vi "main.vi"() -> ()   [LabVIEW 2024]
uses:
  main_state.ctl
  server_state.ctl
panel:
  out "Your IP":string
  in  "Cluster":T1
  in  "stop":bool
  in  "host":bool
  in  "join":bool
  in  "send":bool
  out "chat":string
  in  "message":string
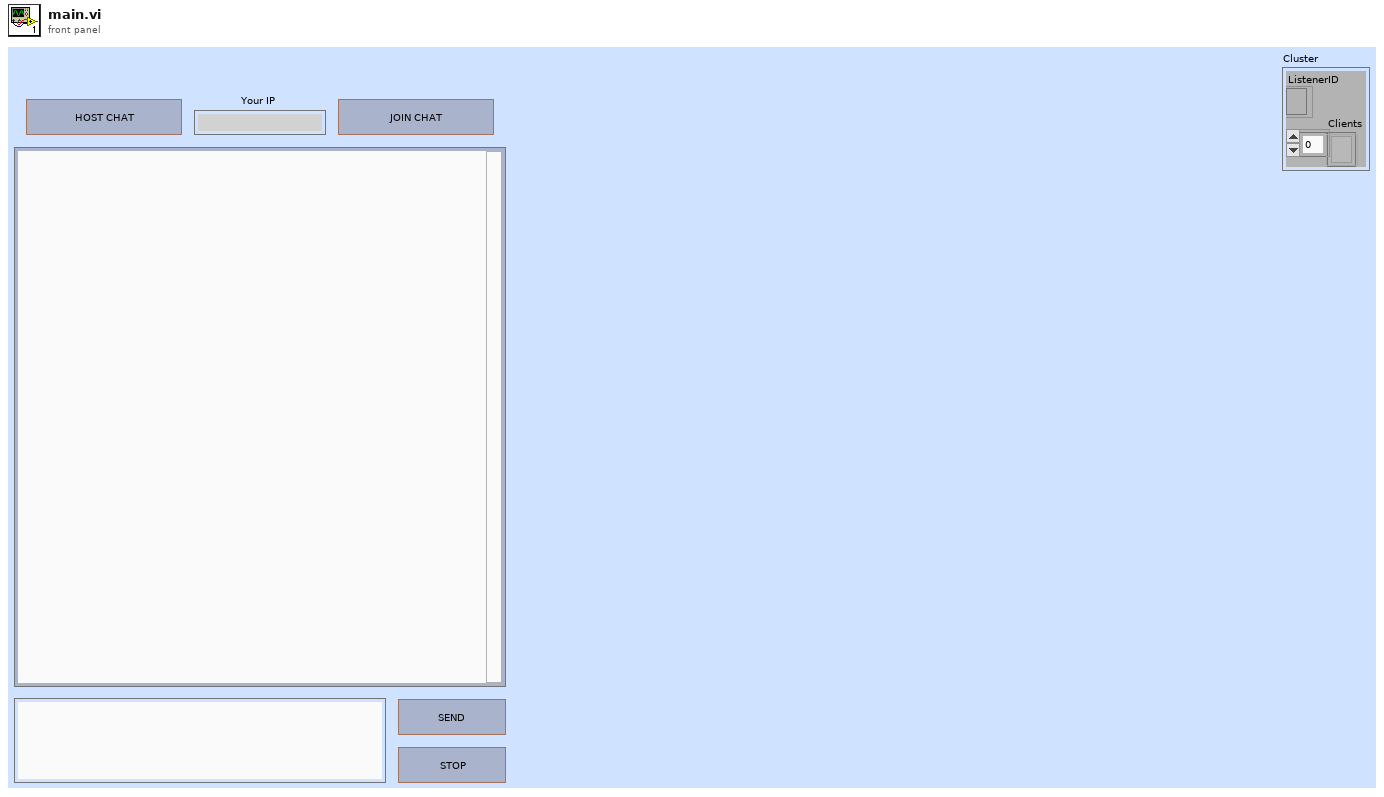
[diagram p1: front panel]
types:
  T1 = cluster{"ListenerID":refnum<k5>, "Clients":refnum<k5>[]}
  T2 = typedef "main_state.ctl" = enum16{"init", "idle", "client", "server", "stop"}
  T3 = typedef "server_state.ctl" = enum16{"Init", "Connect", "Data", "Stop"}
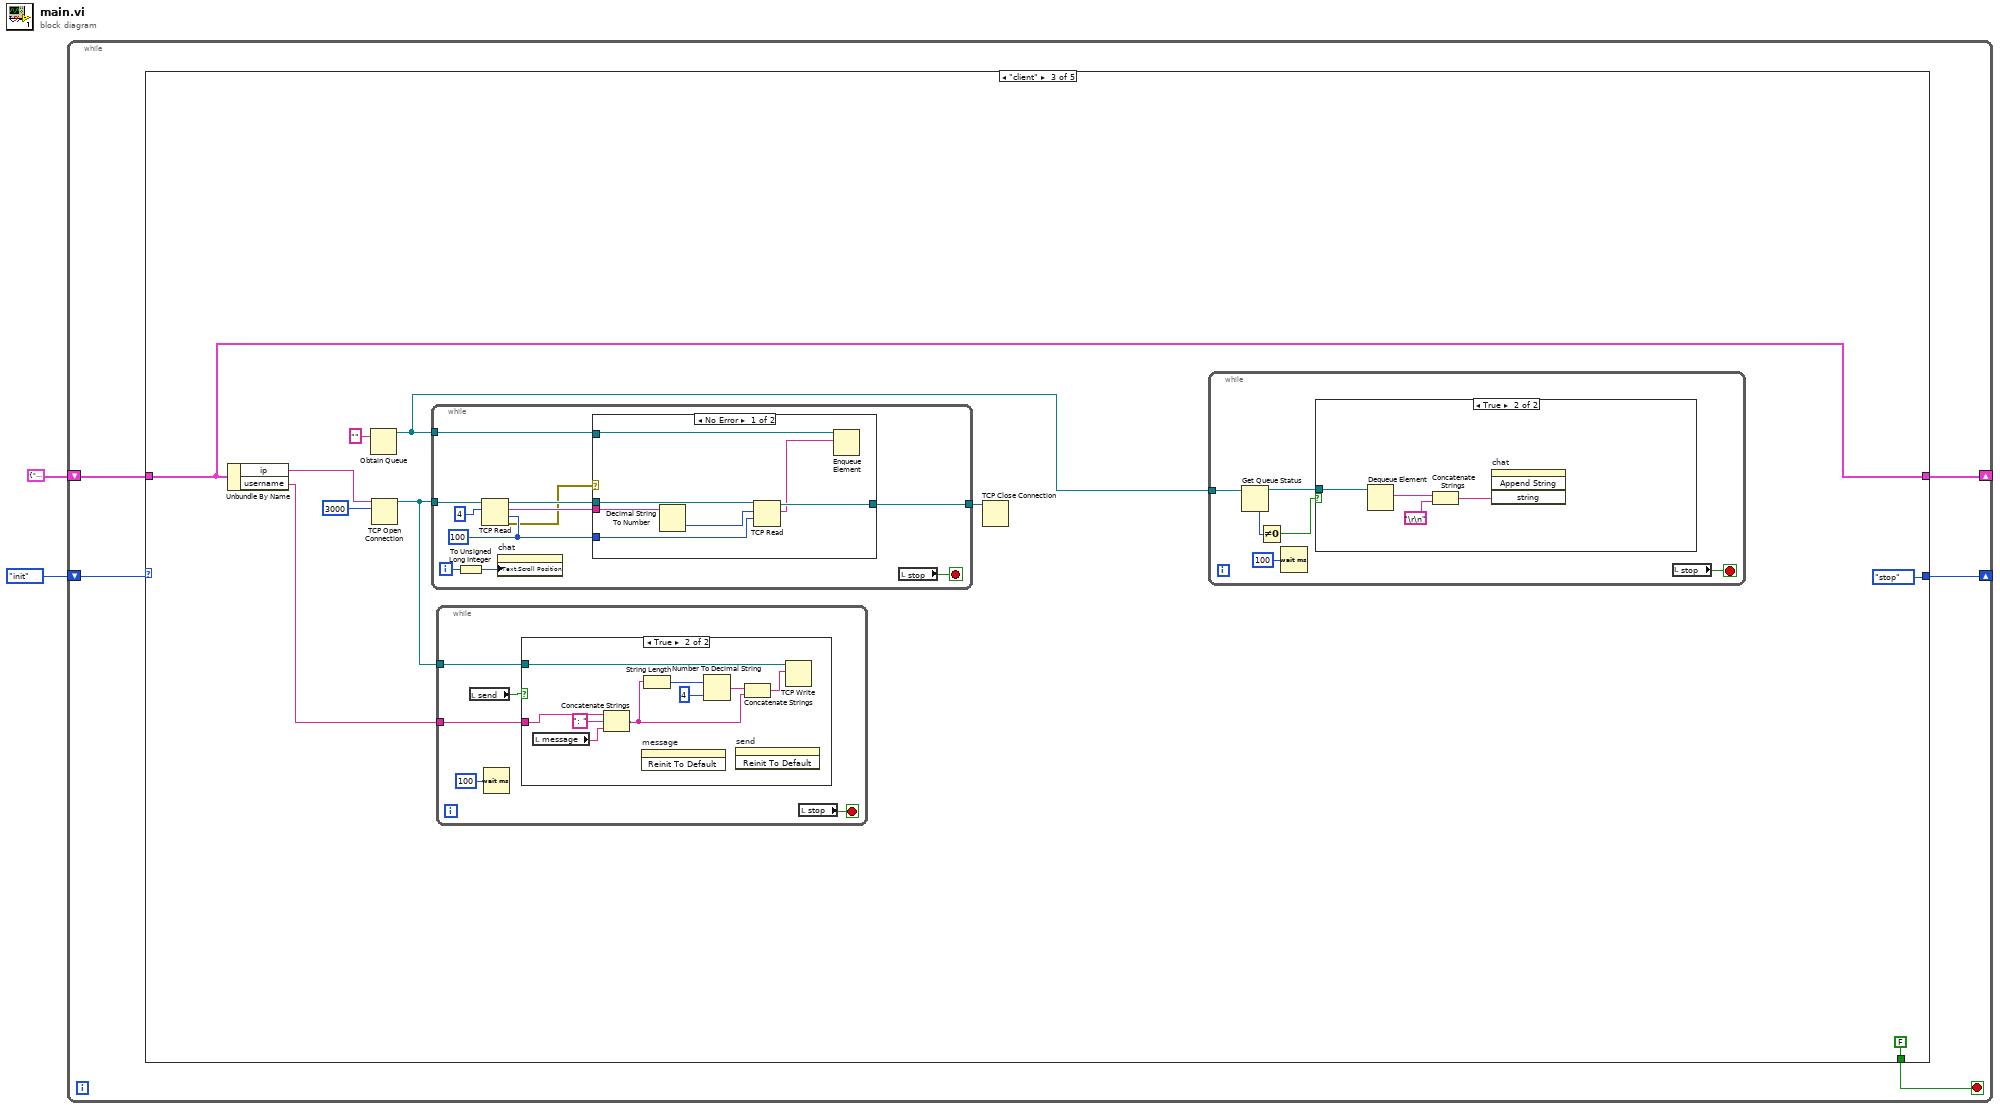
[diagram p0: block diagram]
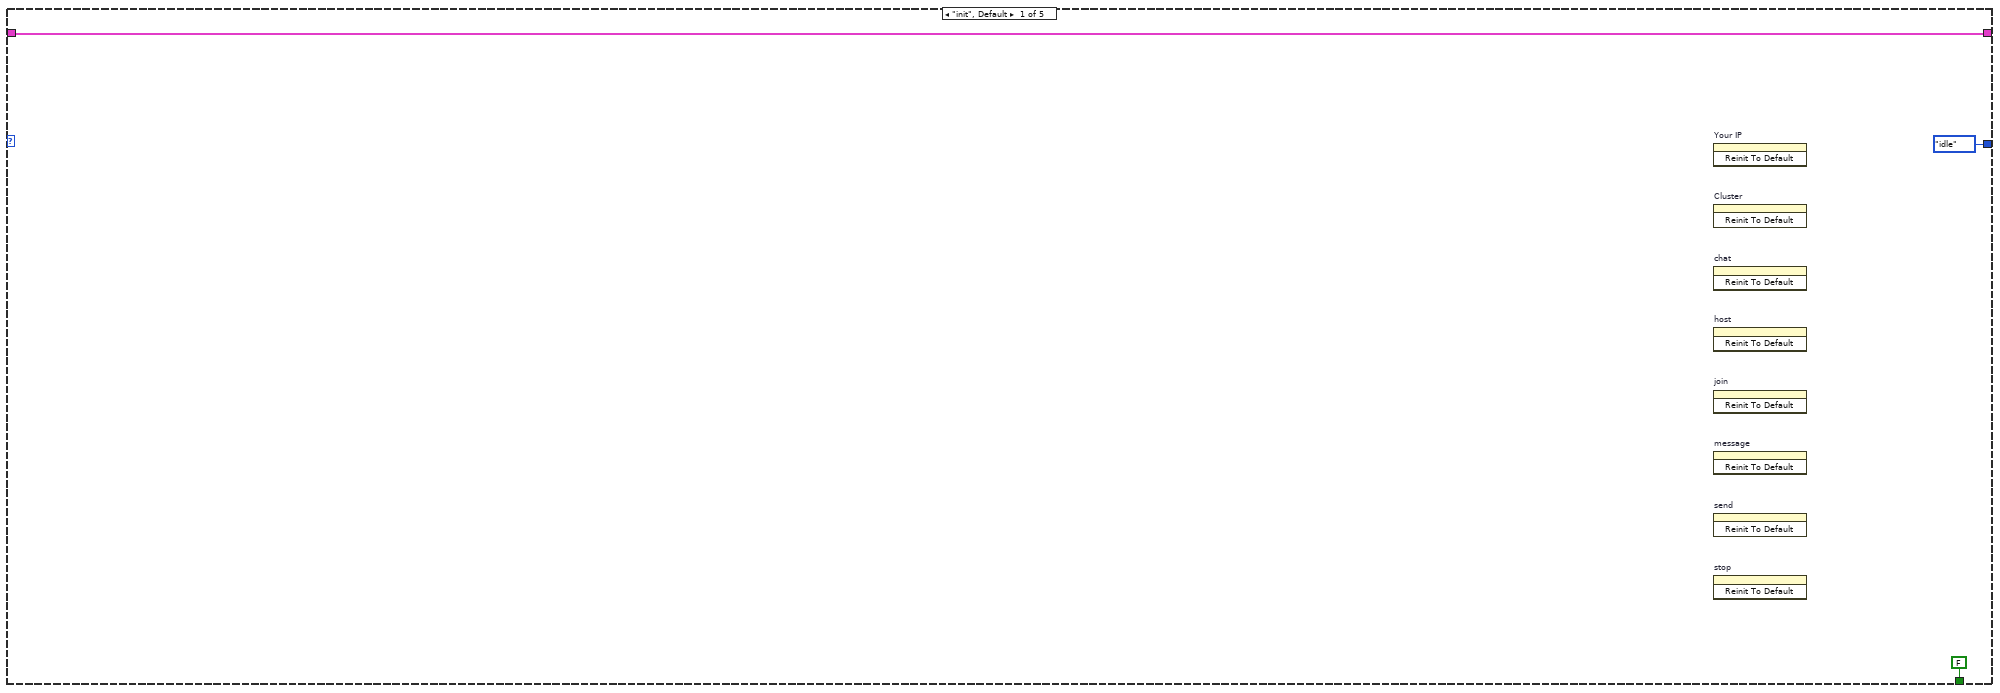
[diagram p2: hidden frame]
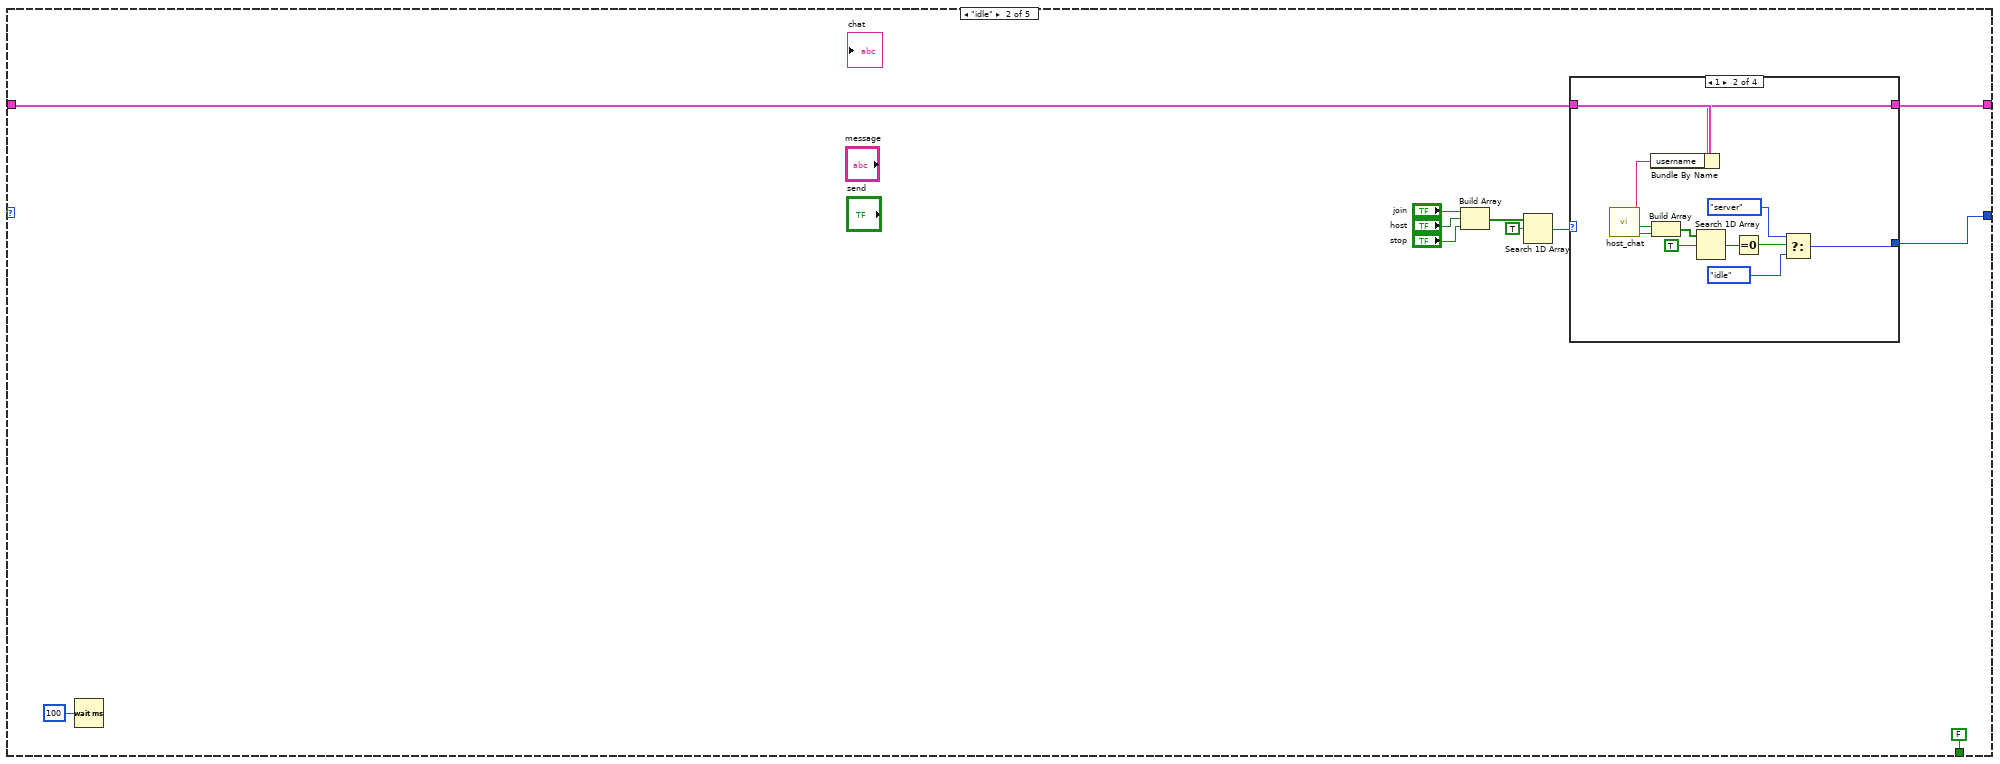
[diagram p3: hidden frame]
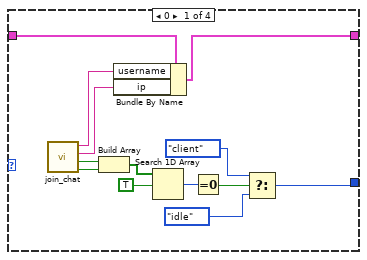
[diagram p4: hidden frame]
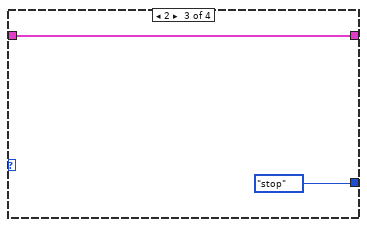
[diagram p5: hidden frame]
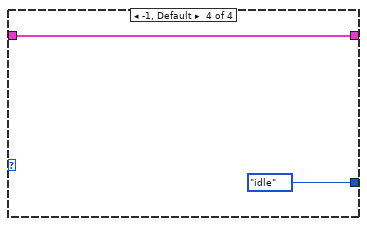
[diagram p6: hidden frame]
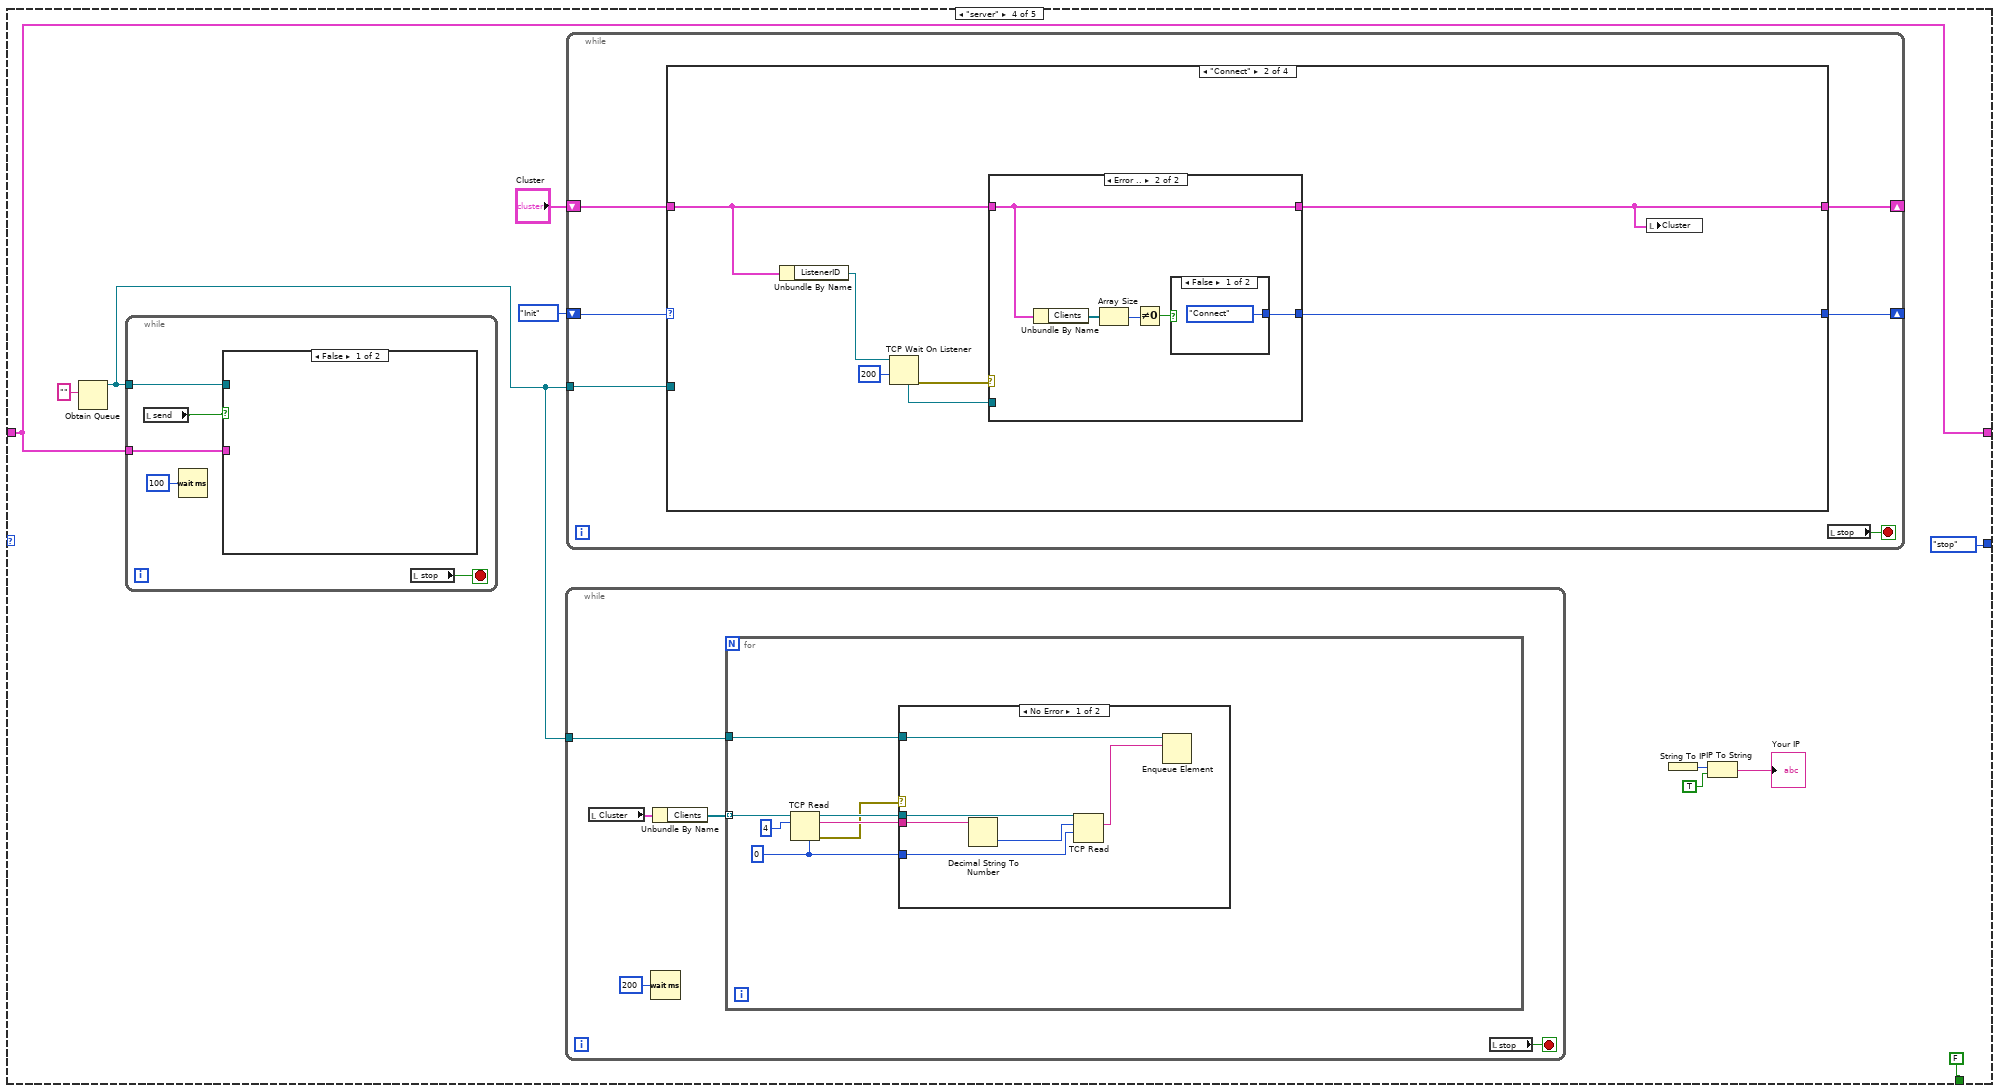
[diagram p10: hidden frame]
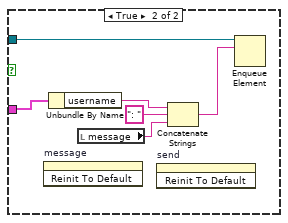
[diagram p12: hidden frame]
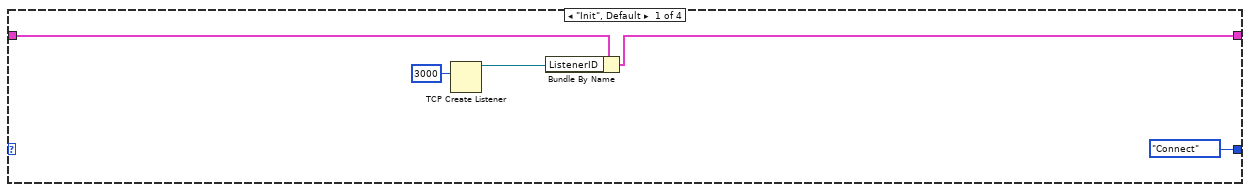
[diagram p13: hidden frame]
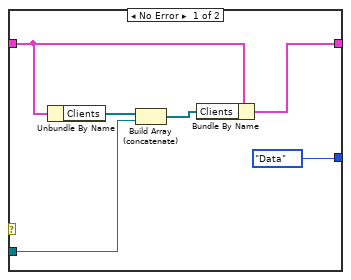
[diagram p14: hidden frame]
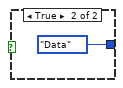
[diagram p15: hidden frame]
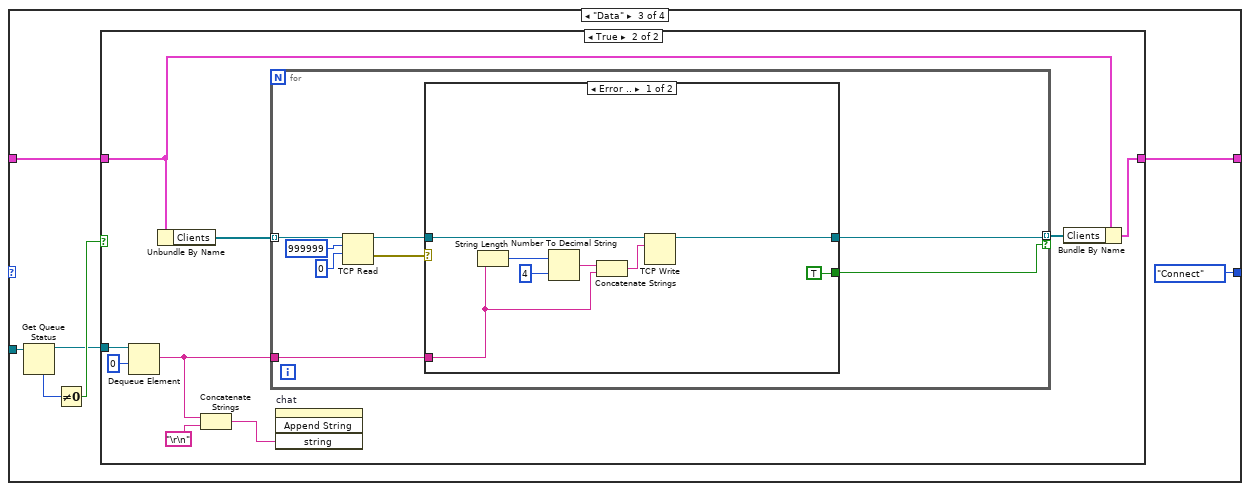
[diagram p16: hidden frame]
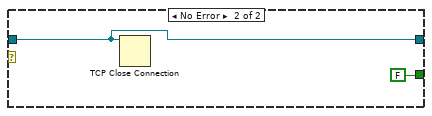
[diagram p18: hidden frame]
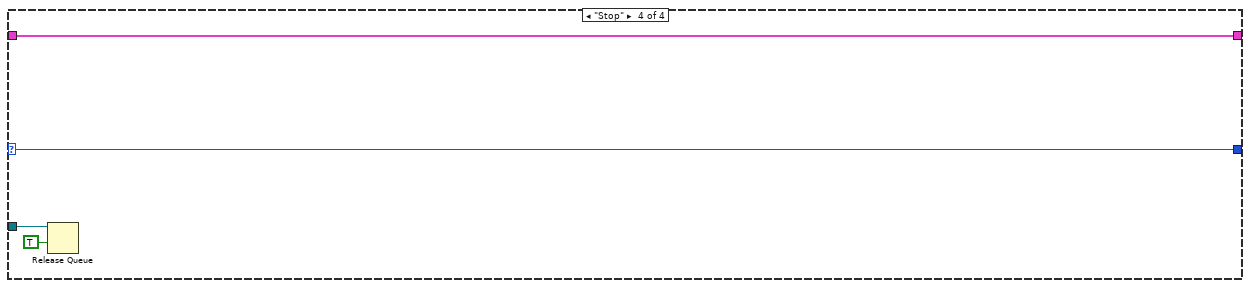
[diagram p19: hidden frame]
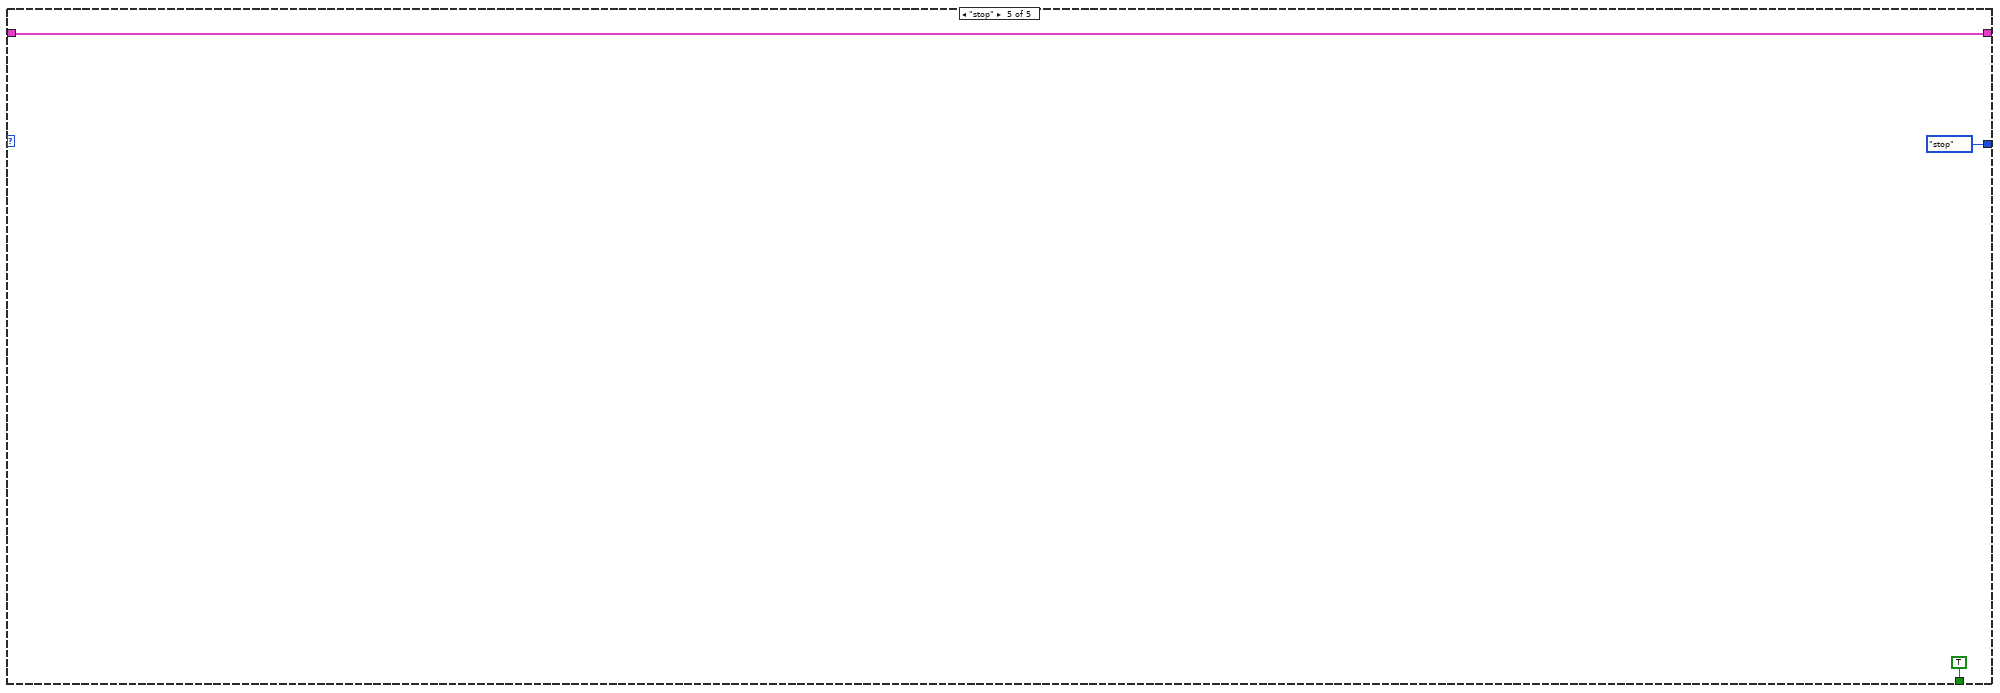
[diagram p20: hidden frame]
diagram:
  n1 = while {
    shift-right: [w5] -> _
    shift-left: main_state."init" ("Enum") -> [w6]
    shift-right: [w3] -> _
    shift-left: cluster{"ip":string, "username":string} {"ip"="", "username"=""} -> [w4]
    stop <- w7 stop-if-true
    n2 = case shown="\"client\"" w6 {
      tunnel: [FALSE FALSE FALSE FALSE TRUE] -> w7
      tunnel: [main_state."idle" ("Enum") w13 main_state."stop" ("Enum") main_state."stop" ("Enum") main_state."stop" ("Enum")] -> w5
      tunnel: w4 -> [w8 w12 w55 w107 w213]
      tunnel: [w8 w11 w55 w107 w213] -> w3
      frame "init", Default {
        n3 = invoke on="Your IP" class="Str" method="Reinit To Default"() -> ()  [unwired: 3 in, 3 out]
        n4 = invoke on="Cluster" class="Clust (strict)" method="Reinit To Default"() -> ()  [unwired: 3 in, 3 out]
        n5 = invoke on="chat" class="Str" method="Reinit To Default"() -> ()  [unwired: 3 in, 3 out]
        n6 = invoke on="host" class="Bool" method="Reinit To Default"() -> ()  [unwired: 3 in, 3 out]
        n7 = invoke on="join" class="Bool" method="Reinit To Default"() -> ()  [unwired: 3 in, 3 out]
        n8 = invoke on="message" class="Str" method="Reinit To Default"() -> ()  [unwired: 3 in, 3 out]
        n9 = invoke on="send" class="Bool (strict)" method="Reinit To Default"() -> ()  [unwired: 3 in, 3 out]
        n10 = invoke on="stop" class="Bool (strict)" method="Reinit To Default"() -> ()  [unwired: 3 in, 3 out]
      }
      frame "idle" {
        n11 = Wait (ms)(milliseconds to wait=u32 100) -> ()  [unwired: 1 out]
        n12 = Build Array("join", "host", "stop") -> (w17:bool[])
        n13 = Search 1D Array(1D array=w17, element=TRUE) -> (index of element=w15:i32)  [unwired: 1 in]
        n14 = case shown="1" w15 {
          tunnel: [w26 w38 main_state."stop" ("Enum") main_state."idle" ("Enum")] -> w13
          tunnel: w12 -> [w25 w37 w47 w49]
          tunnel: [w24 w36 w47 w49] -> w11
          frame 0 {
            n15 = call "join_chat.vi"() -> ("username"=w23:string, "ip"=w22:string, "join"=w33:bool, "cancel"=w32:bool)  [unwired: 1 in]
            n16 = Build Array(w33, w32) -> (w31:bool[])
            n17 = Bundle By Name(cluster=w25, "username"=w23, "ip"=w22) -> (w24:cluster{"ip":string, "username":string})
            n18 = Search 1D Array(1D array=w31, element=TRUE) -> (index of element=w30:i32)  [unwired: 1 in]
            n19 = Equal To 0?(x=w30) -> (x = 0?=w27:bool)
            n20 = Select(t=main_state."client" ("Enum"), s=w27, f=main_state."idle" ("Enum")) -> (s? t:f=w26:T2)
          }
          frame 1 {
            n21 = call "host_chat.vi"() -> ("cancel"=w43:bool, "host"=w44:bool, "username"=w35:string)  [unwired: 9 in]
            n22 = Bundle By Name(cluster=w37, "username"=w35) -> (w36:cluster{"ip":string, "username":string})
            n23 = Build Array(w44, w43) -> (w46:bool[])
            n24 = Search 1D Array(1D array=w46, element=TRUE) -> (index of element=w42:i32)  [unwired: 1 in]
            n25 = Equal To 0?(x=w42) -> (x = 0?=w41:bool)
            n26 = Select(t=main_state."server" ("Enum"), s=w41, f=main_state."idle" ("Enum")) -> (s? t:f=w38:T2)
          }
          frame 2 {
          }
          frame -1, Default {
          }
        }
      }
      frame "client" {
        n27 = Unbundle By Name(w55) -> ("ip"=w56:string, "username"=w54:string)
        n28 = Obtain Queue(element data type="") -> (queue out=w51:refnum<queue>)  [unwired: 4 in, 2 out]
        n29 = TCP Open Connection(address=w56, remote port or service name=u16 3000) -> (connection ID=w52:refnum<k5>)  [unwired: 1 in, 3 out]
        n30 = while {
          tunnel: w52 -> [w69]
          tunnel: [w71] -> w53
          tunnel: w51 -> [w64]
          i -> [w65]
          stop <- w62 stop-if-true
          w70 = 100 ("timeout ms (25000)")
          n31 = To Unsigned Long Integer(number=w65) -> (unsigned 32bit integer=w63:u32)
          n32 = TCP Read(connection ID=w69, bytes to read=4, 9:w70) -> (connection ID out=w67:refnum<k5>, data out=w66:string, error out=w61:errorcluster)  [unwired: 1 in, 1 out]
          n33 = property on="chat" class="Str"("Text.Scroll Position"=w63) -> ()  [unwired: 2 in, 2 out]
          n34 = case shown="No Error" w61 {
            tunnel: [w78 w79] -> w71
            tunnel: w70 -> [w77 _]
            tunnel: w67 -> [w76 w79]
            tunnel: w66 -> [w75 _]
            tunnel: w64 -> [w72 _]
            frame No Error {
              n35 = Decimal String To Number(string=w75) -> (number=w74:i32)  [unwired: 2 in, 1 out]
              n36 = TCP Read(connection ID=w76, bytes to read=w74, 9:w77) -> (connection ID out=w78:refnum<k5>, data out=w73:string)  [unwired: 1 in, 2 out]
              n37 = Enqueue Element(queue=w72, element=w73) -> ()  [unwired: 2 in, 3 out]
            }
            frame Error {
            }
          }
          n38 = local read "stop"() -> (w62:bool)
        }
        n39 = while {
          tunnel: w52 -> [w83]
          tunnel: w54 -> [w80]
          stop <- w81 stop-if-true
          n40 = local read "send"() -> (w82:bool)
          n41 = Wait (ms)(milliseconds to wait=u32 100) -> ()  [unwired: 1 out]
          n42 = case shown="True" w82 {
            tunnel: w83 -> [_ w89]
            tunnel: w80 -> [_ w86]
            frame False {
            }
            frame True {
              n43 = local read "message"() -> (w87:string)
              n44 = Concatenate Strings(w86, ": ", w87) -> (w85:string)
              n45 = invoke on="message" class="Str" method="Reinit To Default"() -> ()  [unwired: 3 in, 3 out]
              n46 = String Length(string=w85) -> (length=w91:i32)
              n47 = Number To Decimal String(number=w91, width (-)=i16 4) -> (decimal integer string=w93:string)
              n48 = invoke on="send" class="Bool (strict)" method="Reinit To Default"() -> ()  [unwired: 3 in, 3 out]
              n49 = Concatenate Strings(w93, w85) -> (w92:string)
              n50 = TCP Write(connection ID=w89, data in=w92) -> ()  [unwired: 2 in, 3 out]
            }
          }
          n51 = local read "stop"() -> (w81:bool)
        }
        n52 = TCP Close Connection(connection ID=w53) -> ()  [unwired: 1 in, 3 out]
        n53 = while {
          tunnel: w51 -> [w97]
          stop <- w94 stop-if-true
          n54 = Get Queue Status(queue=w97) -> (queue out=w96:refnum<queue>, # elements in queue=w99:i32)  [unwired: 2 in, 6 out]
          n55 = Not Equal To 0?(x=w99) -> (x != 0?=w98:bool)
          n56 = Wait (ms)(milliseconds to wait=u32 100) -> ()  [unwired: 1 out]
          n57 = case shown="True" w98 {
            tunnel: w96 -> [_ w103]
            frame False {
            }
            frame True {
              n58 = Dequeue Element(queue=w103) -> (element=w101:string)  [unwired: 2 in, 3 out]
              n59 = Concatenate Strings(w101, "\r\n") -> (w100:string)
              n60 = invoke on="chat" class="Str" method="Append String"("string"=w100) -> ()  [unwired: 3 in, 4 out]
            }
          }
          n61 = local read "stop"() -> (w94:bool)
        }
      }
      frame "server" {
        n62 = Obtain Queue(element data type="" ("name (unnamed)")) -> (queue out=w111:refnum<queue>)  [unwired: 4 in, 2 out]
        n63 = while {
          tunnel: w111 -> [w136]
          tunnel: w107 -> [w133]
          stop <- w132 stop-if-true
          n64 = local read "send"() -> (w134:bool)
          n65 = Wait (ms)(milliseconds to wait=u32 100) -> ()  [unwired: 1 out]
          n66 = case shown="False" w134 {
            tunnel: w136 -> [_ w142]
            tunnel: w133 -> [_ w138]
            frame False {
            }
            frame True {
              n67 = invoke on="message" class="Str" method="Reinit To Default"() -> ()  [unwired: 3 in, 3 out]
              n68 = Unbundle By Name(w138) -> ("username"=w139:string)
              n69 = local read "message"() -> (w141:string)
              n70 = invoke on="send" class="Bool (strict)" method="Reinit To Default"() -> ()  [unwired: 3 in, 3 out]
              n71 = Concatenate Strings(w139, ": ", w141) -> (w137:string)
              n72 = Enqueue Element(queue=w142, element=w137) -> ()  [unwired: 2 in, 3 out]
            }
          }
          n73 = local read "stop"() -> (w132:bool)
        }
        n74 = while {
          tunnel: w111 -> [w117]
          stop <- w114 stop-if-true
          n75 = local read "Cluster"() -> (w115:T1)
          n76 = Wait (ms)(milliseconds to wait=u32 200) -> ()  [unwired: 1 out]
          n77 = Unbundle By Name(w115) -> ("Clients"=w118:refnum<k5>[])
          n78 = for {
            tunnel: w118 -> [w121] mode=indexing
            tunnel: w117 -> [w120]
            w125 = 0 ("timeout ms (25000)")
            n79 = TCP Read(connection ID=w121, bytes to read=4, 9:w125) -> (connection ID out=w123:refnum<k5>, data out=w122:string, error out=w119:errorcluster)  [unwired: 1 in, 1 out]
            n80 = case shown="No Error" w119 {
              tunnel: w125 -> [w131 _]
              tunnel: w123 -> [w130 _]
              tunnel: w122 -> [w129 _]
              tunnel: w120 -> [w126 _]
              frame No Error {
                n81 = Decimal String To Number(string=w129) -> (number=w128:i32)  [unwired: 2 in, 1 out]
                n82 = TCP Read(connection ID=w130, bytes to read=w128, 9:w131) -> (data out=w127:string)  [unwired: 1 in, 3 out]
                n83 = Enqueue Element(queue=w126, element=w127) -> ()  [unwired: 2 in, 3 out]
              }
              frame Error {
              }
            }
          }
          n84 = local read "stop"() -> (w114:bool)
        }
        n85 = while {
          shift-right: [w145] -> _
          shift-left: server_state."Init" ("Enum") -> [w148]
          shift-right: [w146] -> _
          shift-left: "Cluster" -> [w147]
          tunnel: w111 -> [w144]
          stop <- w143 stop-if-true
          n86 = case shown="\"Connect\"" w148 {
            selector: w148 -> [_ _ _ w211]
            tunnel: w147 -> [w152 w158 w179 w212]
            tunnel: [w151 w154 w180 w212] -> w146
            tunnel: [server_state."Connect" ("Enum") w155 server_state."Connect" ("Enum") w211] -> w145
            tunnel: w144 -> [_ _ w177 w210]
            frame "Init", Default {
              n87 = TCP Create Listener(10:u16 3000 ("port")) -> (3:w150:refnum<k5>)  [unwired: 4 in, 2 out]
              n88 = Bundle By Name(cluster=w152, "ListenerID"=w150) -> (w151:T1)
            }
            frame "Connect" {
              n89 = Unbundle By Name(w158) -> ("ListenerID"=w159:refnum<k5>)
              n90 = TCP Wait On Listener(9:200 ("timeout ms (wait forever: -1)"), 11:w159) -> (0:w156:errorcluster, 4:w157:refnum<k5>)  [unwired: 2 in, 3 out]
              n91 = case shown="Error .." w156 {
                tunnel: w158 -> [w166 w171]
                tunnel: w157 -> [w163 _]
                tunnel: [w162 w171] -> w154
                tunnel: [server_state."Data" ("Enum") w167] -> w155
                frame No Error {
                  n92 = Unbundle By Name(w166) -> ("Clients"=w165:refnum<k5>[])
                  n93 = Build Array (concatenate)(w165, w163) -> (w164:refnum<k5>[])
                  n94 = Bundle By Name(cluster=w166, "Clients"=w164) -> (w162:T1)
                }
                frame Error {
                  n95 = Unbundle By Name(w171) -> ("Clients"=w170:refnum<k5>[])
                  n96 = Array Size(array=w170) -> (size(s)=w169:i32)
                  n97 = Not Equal To 0?(x=w169) -> (x != 0?=w168:bool)
                  n98 = case shown="False" w168 {
                    tunnel: [server_state."Connect" ("Enum") server_state."Data" ("Enum")] -> w167
                    frame False {
                    }
                    frame True {
                    }
                  }
                }
              }
              n99 = local write "Cluster"(w154) -> ()
            }
            frame "Data" {
              n100 = Get Queue Status(queue=w177) -> (queue out=w174:refnum<queue>, # elements in queue=w176:i32)  [unwired: 2 in, 6 out]
              n101 = Not Equal To 0?(x=w176) -> (x != 0?=w175:bool)
              n102 = case shown="True" w175 {
                tunnel: [w181 w189] -> w180
                tunnel: w179 -> [w181 w188]
                tunnel: w174 -> [_ w186]
                frame False {
                }
                frame True {
                  n103 = Dequeue Element(queue=w186, timeout in ms (-1)=0) -> (element=w182:string)  [unwired: 1 in, 3 out]
                  n104 = Unbundle By Name(w188) -> ("Clients"=w190:refnum<k5>[])
                  n105 = Concatenate Strings(w182, "\r\n") -> (w183:string)
                  n106 = for {
                    tunnel: w190 -> [w198] mode=indexing
                    tunnel: [w195] -> w187 mode=indexing if=w194
                    tunnel: w182 -> [w191]
                    n107 = TCP Read(connection ID=w198, bytes to read=999999, 9:0 ("timeout ms (25000)")) -> (connection ID out=w196:refnum<k5>, error out=w193:errorcluster)  [unwired: 2 in, 1 out]
                    n108 = case shown="Error .." w193 {
                      tunnel: w196 -> [w206 w208]
                      tunnel: [w205 w208] -> w195
                      tunnel: [TRUE FALSE] -> w194
                      tunnel: w191 -> [w199 _]
                      frame Error {
                        n109 = String Length(string=w199) -> (length=w203:i32)
                        n110 = Number To Decimal String(number=w203, width (-)=i16 4) -> (decimal integer string=w200:string)
                        n111 = Concatenate Strings(w200, w199) -> (w201:string)
                        n112 = TCP Write(connection ID=w206, data in=w201) -> (connection ID out=w205:refnum<k5>)  [unwired: 2 in, 2 out]
                      }
                      frame No Error {
                        n113 = TCP Close Connection(connection ID=w208) -> ()  [unwired: 1 in, 3 out]
                      }
                    }
                  }
                  n114 = invoke on="chat" class="Str" method="Append String"("string"=w183) -> ()  [unwired: 3 in, 4 out]
                  n115 = Bundle By Name(cluster=w188, "Clients"=w187) -> (w189:T1)
                }
              }
            }
            frame "Stop" {
              n116 = Release Queue(queue=w210, force destroy? (F)=TRUE) -> ()  [unwired: 1 in, 3 out]
            }
          }
          n117 = local read "stop"() -> (w143:bool)
        }
        n118 = String To IP() -> (0:w104:u32)  [unwired: 1 in]
        n119 = IP To String(1:TRUE ("dot notation? (F)"), 2:w104) -> (0:→"Your IP":string)
      }
      frame "stop" {
      }
    }
  }
